vi "Apply Direction.vi"(8 "error in (no error)":errorcluster, 11 "Tool Path in":refnum<class "Tool Path.lvclass">) -> (0 "error out":errorcluster, 3 "Tool Path out":refnum<class "Tool Path.lvclass">)   [LabVIEW 2019, in "Tool Path.lvclass"]
uses:
  Tool Path.lvclass
  Settings/ObjectSettings/ObjectSettings.lvclass/ObjectSettings.ctl
  Settings/Path Settings/Path Settings.lvclass
  C:/Users/Albro/Documents/GitHub/AFM-Lithography/lvsrc/Classes/Settings/ObjectSettings/ObjectSettings.lvclass
  Settings/ObjectSettings/ObjectSettings.lvclass
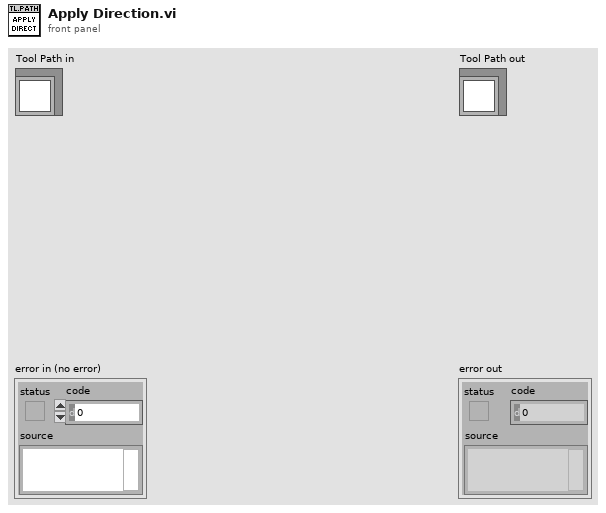
[diagram p1: front panel]
types:
  T1 = typedef "PathCommands.lvclass/Point.ctl" = cluster{"X":dbl, "Y":dbl}
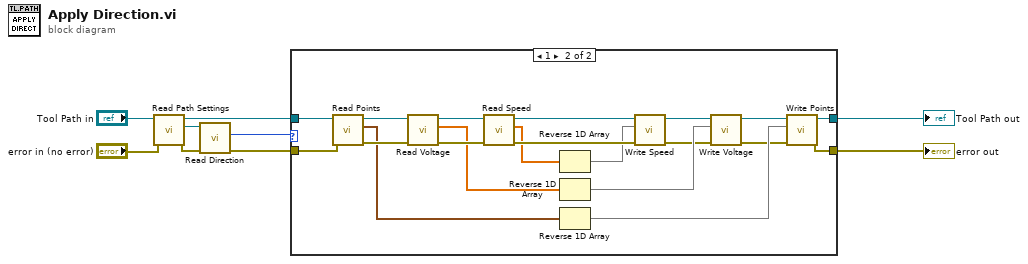
[diagram p0: block diagram]
diagram:
  n1 = call-dynamic "Read Path Settings.vi"("error in (no error)"="error in (no error)", "Tool Path in"="Tool Path in") -> ("error out"=w4:errorcluster, "Path Settings.lvclass"=w6:refnum<class "Path Settings.lvclass">, "Tool Path out"=w7:refnum<class "Tool Path.lvclass">)  [unwired: 7 in]
  n2 = call "Read Direction.vi"("error in (no error)"=w4, "ObjectSettings in"=w6) -> ("error out"=w3:errorcluster, "Direction"=w1:u16)  [unwired: 7 in, 1 out]
  n3 = case shown="1" w1 {
    tunnel: [w11 w16] -> w9
    tunnel: w7 -> [w11 w28]
    tunnel: w3 -> [w10 w27]
    tunnel: [w10 w15] -> w2
    frame 0, Default {
    }
    frame 1 {
      n4 = call-dynamic "Read Points.vi"("error in (no error)"=w27, "Tool Object in"=w28) -> ("error out"=w26:errorcluster, "Points"=w12:T1[], "Tool Object out"=w31:refnum<class "Tool Path.lvclass">)  [unwired: 7 in]
      n5 = call-dynamic "Read Voltage.vi"("error in (no error)"=w26, "Tool Object in"=w31) -> ("error out"=w25:errorcluster, "Voltage"=w21:dbl[], "Tool Object out"=w30:refnum<class "Tool Path.lvclass">)  [unwired: 7 in]
      n6 = call-dynamic "Read Speed.vi"("error in (no error)"=w25, "Tool Object in"=w30) -> ("error out"=w24:errorcluster, "Speed"=w23:dbl[], "Tool Object out"=w29:refnum<class "Tool Path.lvclass">)  [unwired: 7 in]
      n7 = Reverse 1D Array(array=w23) -> (reversed array=w22:dbl[])
      n8 = Reverse 1D Array(array=w21) -> (reversed array=w19:dbl[])
      n9 = Reverse 1D Array(array=w12) -> (reversed array=w18:T1[])
      n10 = call-dynamic "Write Speed.vi"("error in (no error)"=w24, "Speed"=w22, "Tool Object in"=w29) -> ("error out"=w13:errorcluster, "Tool Object out"=w20:refnum<class "Tool Path.lvclass">)  [unwired: 7 in]
      n11 = call-dynamic "Write Voltage.vi"("error in (no error)"=w13, "Voltage"=w19, "Tool Object in"=w20) -> ("error out"=w14:errorcluster, "Tool Object out"=w17:refnum<class "Tool Path.lvclass">)  [unwired: 7 in]
      n12 = call-dynamic "Write Points.vi"("error in (no error)"=w14, "Points"=w18, "Tool Object in"=w17) -> ("error out"=w15:errorcluster, "Tool Object out"=w16:refnum<class "Tool Path.lvclass">)  [unwired: 7 in]
    }
  }
  "error out" <- w2
  "Tool Path out" <- w9
